vi "Wojtyna_Target_C_1.vi"   [LabVIEW 2020]
uses:
  <vilib>/Platform/TimedLoop/XDataNode/timing_clust.ctl
  <vilib>/Platform/TimedLoop/XDataNode/nitl_modes.ctl
  <vilib>/Platform/TimedLoop/XDataNode/wakeup.ctl
  <vilib>/platform/TimedLoop/XDataNode/XDataNode.xnode
  <vilib>/Platform/TimedLoop/XDataNode/XDNodeRunTimeDep.lvlib
types:
  T1 = typedef "XDNodeRunTimeDep.lvlib/timing_clust.ctl" = cluster{"Expected End [f-1]":u64, "Actual End [f-1]":u64, "Finished Late? [f-1]":bool, "Expected End [i-1]":u64, "Actual End [i-1]":u64, "Finished Late? [i-1]":bool, "Expected Start [i]":u64, "Actual Start [i]":u64, "Expected Start [f]":u64, "Actual Start [f]":u64, "Source Name":string, "Structure Name":string, "Period":i64, "Deadline":i64, "Offset":i64, "Start":i64, "Priority":i32, "Timeout":i32, "Mode":T2, "Wakeup Reason":T3, "Error":errorcluster, "Source Type":string, "Secondary Source Type":string, "Global End Time":u64, "Global Start Time":u64, "Frame Duration":u64, "Iteration Duration":u64, "Assigned CPU":i32, "I/O Scan Engine Mode":u32}
  T2 = typedef "XDNodeRunTimeDep.lvlib/nitl_modes.ctl" = enum32{"No Change", "Process missed periods, maintain original phase", "Discard missed periods, maintain original phase", "Process missed periods, ignore original phase", "Discard missed periods, ignore original phase"}
  T3 = typedef "XDNodeRunTimeDep.lvlib/wakeup.ctl" = enum32{"Normal", "Aborted", "Asynchronous wakeup", "Timing source error", "Timed loop error", "Timeout"}
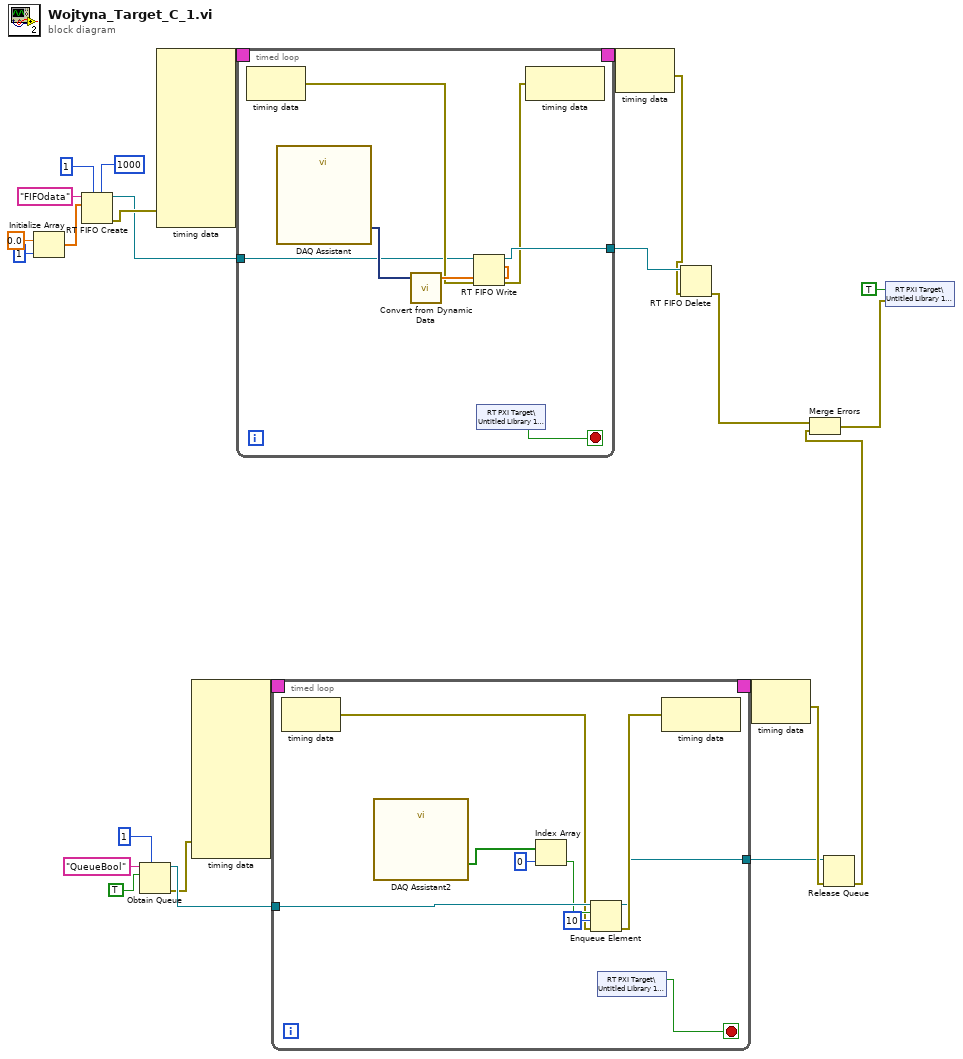
[diagram p0: block diagram]
diagram:
  n1 = Initialize Array(0.0 ("element"), 1 ("dimension size")) -> (w20:dbl[])
  n2 = RT FIFO Create(0:"FIFOdata" ("name (unnamed)"), 1:w20, 4:u32 1 ("size (10)"), 6:u32 1000 ("elements in array (1)")) -> (8:w1:refnum<k33>, 11:w13:errorcluster)  [unwired: 4 in, 1 out]
  n3 = Obtain Queue(max queue size (-1, unlimited)=1, name (unnamed)="QueueBool", element data type=TRUE) -> (queue out=w8:refnum<queue>, error out=w5:errorcluster)  [unwired: 2 in, 1 out]
  n4 = node-c288(w13) -> (w25:T1)  [unwired: 9 in]
  n5 = node-c288(w5) -> (w23:T1)  [unwired: 9 in]
  n6 = timed-loop {
    timing: w25 -> [_]
    timing-out: [_] -> w24
    tunnel: [w30] -> w15
    tunnel: w1 -> [w26]
    stop <- w29 stop-if-true
    n7 = node-c288() -> (w27:errorcluster)  [unwired: 1 in]
    n8 = call "DAQ Assistant"() -> ("data"=w32:dynamicdata)  [unwired: 17 in, 2 out]
    n9 = call "Convert from Dynamic Data"("Dynamic Data Type"=w32) -> ("Array"=w31:dbl[])  [unwired: 3 in]
    n10 = RT FIFO Write(0:w26, 1:w31, 3:w27) -> (8:w30:refnum<k33>, 11:w28:errorcluster)  [unwired: 2 in, 2 out]
    n11 = shared-variable "RT PXI Target\\Untitled Library 1.lvlib\\Stop"() -> (w29:bool)  [unwired: 1 in, 1 out]
    n12 = node-c288(w28) -> ()  [unwired: 1 out]
  }
  n13 = timed-loop {
    timing: w23 -> [_]
    timing-out: [_] -> w22
    tunnel: w8 -> [w46]
    tunnel: [w40] -> w6
    stop <- w38 stop-if-true
    n14 = node-c288() -> (w39:errorcluster)  [unwired: 1 in]
    n15 = call "DAQ Assistant2"() -> ("data"=w45:bool[])  [unwired: 17 in, 2 out]
    n16 = Index Array(array=w45, index=0) -> (element=w43:bool)
    n17 = Enqueue Element(queue=w46, element=w43, timeout in ms (-1)=10, error in (no error)=w39) -> (queue out=w40:refnum<queue>, error out=w41:errorcluster)  [unwired: 1 out]
    n18 = shared-variable "RT PXI Target\\Untitled Library 1.lvlib\\Stop"() -> (w38:bool)  [unwired: 1 in, 1 out]
    n19 = node-c288(w41) -> ()  [unwired: 1 out]
  }
  n20 = node-c288(w24) -> (w14:errorcluster)
  n21 = RT FIFO Delete(0:w15, 3:w14) -> (11:w3:errorcluster)  [unwired: 1 in]
  n22 = node-c288(w22) -> (w7:errorcluster)
  n23 = Release Queue(queue=w6, error in (no error)=w7) -> (error out=w2:errorcluster)  [unwired: 1 in, 2 out]
  n24 = Merge Errors(w3, w2) -> (w4:errorcluster)
  n25 = shared-variable "RT PXI Target\\Untitled Library 1.lvlib\\Stop"(TRUE ("Stop"), error in=w4) -> ()  [unwired: 1 out]
